vi "SAW.vi"(0 "File or Folder Path":path=path "G:/.shortcut-targets-by-id/0B8-gGFa6hkR4XzJJMDlqZXVKRk0/ansom/Data/MNK/SA40516Jref.20250417/05-Bsweepup", 5 "offset":i32, 7 "length":i32=400, 9 "index":T4={"S21"="S21", "S21 after subtraction"="S21", "S12"="S12", "S22"="S22", "Top gate "="frequency", "Bottom Gate"="frequency", "Local Gate"="frequency", "B/Time"="Magnet", "X axis"="frequency", "Temp"="Magnet Field"}, 11 "stop":bool, 12 "File Type":T3=enum."TDMS", 13 "decimate files":i32=2) -> (10 "Gates and B":T1={"Top gate"=100000000.0, "Bottom Gate"=100000000.0, "Local Gate"=100000000.0, "B"=0.11, "X axis"=100000000.0}, 14 "Comments":string="Device: \r  Device Name: SA40516Jref.20250417\r  Computer: Kholek\r  User: Muqing/Ranjani/Pubudu\r  Instrument: MNK\r  Description: |\r    KTO J Resonator - Reference\r    DC = 7/9 = KH1/2\r    Vbg=AO8=26\r\rExperiment: \r  Time: 2025-04-19T03:04:53\r  Description: |\r    T = 58mK\r    B=0T to 0.2T, 0.0005T step\r    Vbg(AO6) = 0V\r    Power: -19.6 dBm\r    0.1 to 2GHz\r    Vd: 1.3V\r    Id: 9.5mA\r\rSweep: \r- Loop1: [Magnet Field, 0.111000]\r- Loop2: [OFF, 0.000000]\r- Loop3: [OFF, 0.000000]\r- Loop4: [OFF, 0.000000]\r\rWiring: \r- Electrode 7: Lockin 1, I+\r- Electrode 11: Lockin 2, I-\r- Electrode 26: Lockin 8, \r\rLockin: \r  AO: \r  - AO 1: amp = 0.000 mV, DC = 0.000 mV, f = 13.00 Hz, phi = 0.00°, Sine\r  - AO 2: amp = 0.000 mV, DC = 0.000 mV, f = 13.00 Hz, phi = 0.00°, Sine\r  - AO 3: amp = 0.000 mV, DC = 0.000 mV, f = 13.00 Hz, phi = 0.00°, Sine\r  - AO 4: amp = 0.000 mV, DC = 0.000 mV, f = 13.00 Hz, phi = 0.00°, Sine\r  - AO 5: amp = 0.000 mV, DC = 0.000 mV, f = 13.00 Hz, phi = 0.00°, Sine\r  - AO 6: amp = 0.000 mV, DC = 0.000 mV, f = 13.00 Hz, phi = 0.00°, Sine\r  - AO 7: amp = 0.000 mV, DC = 0.000 mV, f = 13.00 Hz, phi = 0.00°, Sine\r  - AO 8: amp = 0.000 mV, DC = 0.000 mV, f = 13.00 Hz, phi = 0.00°, Sine\r  - AO 9: amp = 0.000 mV, DC = 0.000 mV, f = 13.00 Hz, phi = 0.00°, Sine\r  - AO 10: amp = 0.000 mV, DC = 0.000 mV, f = 13.00 Hz, phi = 0.00°, Sine\r  REF: \r  - Lockin 1: f = 13.00 Hz, phi = 0.00°, TC = 0.10 s, order = 2 \r  Sampling: \r  - Fs: 6500.000006\r  - N: 500\r")   [LabVIEW 2020]
uses:
  <userlib>/LevyLab/LV-Data/LV-Data/Typedefs/File Type--enum.ctl
  <userlib>/LevyLab/LV-Data/LV-Data/Typedefs/Dictionary--cluster.ctl
  <vilib>/Analysis/3filter.llb/Filter Passband Type.ctl
  <userlib>/LevyLab/Graph Utilities/graph_utilities.lvclass/graph_utilities.ctl
  <vilib>/Analysis/2dsp.llb/Decimate (single shot, DBL).vi
  <userlib>/LevyLab/XY Utilities/subVIs/Peak Detector (single).vi
  <userlib>/LevyLab/XY Utilities/subVIs/Subtract XY (single).vi
  <userlib>/LevyLab/XY Utilities/Private/X Units.vi
  <userlib>/LevyLab/XY Utilities/Private/X Array Range to Index.vi
  <userlib>/_MGI/1D Array/MGI Interpolate 1D Array Extended.vi
  <vilib>/Utility/error.llb/Error Cluster From Error Code.vi
  <vilib>/Analysis/3filter.llb/Butterworth Filter (DBL).vi
  <userlib>/LevyLab/Graph Utilities/graph_utilities.lvclass
  <userlib>/LevyLab/LV-Data/LV-Data/LV-Data.lvclass
  <vilib>/Analysis/NI_AALPro.lvlib
  <userlib>/LevyLab/XY Utilities/xy_utilities.lvlib
  <vilib>/Analysis/NI_AALBase.lvlib
panel:
  in  "Subtract this":cluster{dbl[], dbl[]}[](graph)=[{array[1601 elements], array[1601 elements]}]
  in  "filter order":i32=1
  in  "low cutoff freq":dbl=0.12500000000000006 format="%0.4f"
  in  "Add filter?":bool
  in  "Convert S21 to WAtts":bool
  out "XY-data out":cluster{"X-array":dbl[], "Y-array":dbl[]}[](array[cluster]) {"Y-array" format="%.2p"; "X-array" format="%.2p"}
  in  "threshold":dbl format="%0.2f"
  in  "width":dbl=3.0 min=3.0
  in  "Width Unit (points)":enum16{"Points", "Data"}(ring)
  out "Peak position vs parameter":cluster{dbl[], dbl[]}[](graph)
  out "S22":dbl[][](graph)
  out "S22 vs f":cluster{dbl[], dbl[]}[](graph)
  out "S12":dbl[][](graph)
  out "S12 vs f":cluster{dbl[], dbl[]}[](graph)
  out "S21 atr sub":dbl[][](graph)
  out "S11 vs f":cluster{dbl[], dbl[]}[](graph)
  out "S21":dbl[][](graph)
  in  "decimating factor":i32=1
  out "S21 vs f":cluster{dbl[], dbl[]}[](graph)
  out "Temp vs Field/Time":cluster{dbl[], dbl[]}[](graph)=[{[0.0001], [0.0]}, {[0.001], [0.001]}, {[0.002], [0.002]}, {[0.003], [0.003]}, {[0.004], [0.004]}, {[0.005], [0.005]}, {[0.006], [0.006]}, {[0.007], [0.007]}, {[0.008], [0.008]}, {[0.009], [0.009000000000000001]}, {[0.01], [0.01]}, {[0.011], [0.011]}, {[0.012], [0.012]}, {[0.013], [0.013000000000000001]}, {[0.014], [0.014]}, {[0.015], [0.015]}, {[0.016], [0.016]}, {[0.017], [0.017]}, {[0.018], [0.018000000000000002]}, {[0.019], [0.019]}, {[0.02], [0.02]}, {[0.021], [0.021]}, {[0.022], [0.022]}, {[0.0231], [0.023]}, {[0.024], [0.024]}, {[0.0251], [0.025]}, {[0.026], [0.026000000000000002]}, {[0.0269], [0.027]}, {[0.0281], [0.028]}, {[0.029], [0.029]}, {[0.03], [0.03]}, {[0.0311], [0.031]}, {[0.032], [0.032]}, {[0.033], [0.033]}, {[0.034], [0.034]}, {[0.035], [0.035]}, {[0.036], [0.036000000000000004]}, {[0.037], [0.037]}, {[0.0375], [0.038]}, {[0.039], [0.039]}, {[0.04], [0.04]}, {[0.041], [0.041]}, {[0.042], [0.042]}, {[0.043], [0.043000000000000003]}, {[0.044], [0.044]}, {[0.045], [0.045]}, {[0.046], [0.046]}, {[0.047], [0.047]}, {[0.048], [0.048]}, {[0.049], [0.049]}, {[0.05], [0.05]}, {[0.051], [0.051000000000000004]}, {[0.052], [0.052000000000000005]}, {[0.0527], [0.053]}, {[0.054], [0.054]}, {[0.055], [0.055]}, {[0.056], [0.056]}, {[0.057], [0.057]}, {[0.058], [0.058]}, {[0.059], [0.059000000000000004]}, {[0.06], [0.06]}, {[0.0611], [0.061]}, {[0.062], [0.062]}, {[0.063], [0.063]}, {[0.064], [0.064]}, {[0.065], [0.065]}, {[0.066], [0.066]}, {[0.0671], [0.067]}, {[0.068], [0.068]}, {[0.069], [0.069]}, {[0.07], [0.07]}, {[0.071], [0.07100000000000001]}, {[0.072], [0.07200000000000001]}, {[0.073], [0.073]}, {[0.074], [0.074]}, {[0.075], [0.075]}, {[0.076], [0.076]}, {[0.077], [0.077]}, {[0.078], [0.078]}, {[0.0791], [0.079]}, {[0.08], [0.08]}, {[0.081], [0.081]}, {[0.082], [0.082]}, {[0.083], [0.083]}, {[0.084], [0.084]}, {[0.085], [0.085]}, {[0.086], [0.08600000000000001]}, {[0.087], [0.08700000000000001]}, {[0.088], [0.088]}, {[0.089], [0.089]}, {[0.0901], [0.09]}, {[0.091], [0.091]}, {[0.092], [0.092]}, {[0.093], [0.093]}, {[0.094], [0.094]}, {[0.095], [0.095]}, {[0.096], [0.096]}, {[0.097], [0.097]}, {[0.098], [0.098]}, {[0.099], [0.099]}, {[0.1], [0.1]}, {[0.1011], [0.101]}, {[0.1019], [0.10200000000000001]}, {[0.103], [0.10300000000000001]}, {[0.104], [0.10400000000000001]}, {[0.105], [0.105]}, {[0.106], [0.106]}, {[0.107], [0.107]}, {[0.108], [0.108]}, {[0.1091], [0.109]}, {[0.11], [0.11]}, {[0.1111], [0.111]}, {[0.1121], [0.112]}, {[0.113], [0.113]}, {[0.114], [0.114]}, {[0.115], [0.115]}, {[0.116], [0.116]}, {[0.117], [0.117]}, {[0.118], [0.11800000000000001]}, {[0.119], [0.11900000000000001]}, {[0.12], [0.12]}, {[0.121], [0.121]}, {[0.122], [0.122]}, {[0.123], [0.123]}, {[0.124], [0.124]}, {[0.125], [0.125]}, {[0.126], [0.126]}, {[0.127], [0.127]}, {[0.128], [0.128]}, {[0.129], [0.129]}, {[0.13], [0.13]}, {[0.131], [0.131]}, {[0.132], [0.132]}, {[0.133], [0.133]}, {[0.134], [0.134]}, {[0.135], [0.135]}, {[0.136], [0.136]}, {[0.137], [0.137]}, {[0.138], [0.138]}, {[0.139], [0.139]}, {[0.14], [0.14]}, {[0.1411], [0.14100000000000001]}, {[0.142], [0.14200000000000002]}, {[0.143], [0.14300000000000002]}, {[0.144], [0.14400000000000002]}, {[0.1451], [0.145]}, {[0.146], [0.146]}, {[0.147], [0.147]}, {[0.1481], [0.148]}, {[0.149], [0.149]}, {[0.15], [0.15]}, {[0.151], [0.151]}, {[0.1521], [0.152]}, {[0.1531], [0.153]}, {[0.154], [0.154]}, {[0.155], [0.155]}, {[0.156], [0.156]}, {[0.157], [0.157]}, {[0.1581], [0.158]}, {[0.159], [0.159]}, {[0.1601], [0.16]}, {[0.161], [0.161]}, {[0.1621], [0.162]}, {[0.163], [0.163]}, {[0.164], [0.164]}, {[0.165], [0.165]}, {[0.166], [0.166]}, {[0.1671], [0.167]}, {[0.168], [0.168]}, {[0.169], [0.169]}, {[0.17], [0.17]}, {[0.171], [0.171]}, {[0.172], [0.17200000000000001]}, {[0.173], [0.17300000000000001]}, {[0.1741], [0.17400000000000002]}, {[0.175], [0.17500000000000002]}, {[0.176], [0.176]}, {[0.177], [0.177]}, {[0.178], [0.178]}, {[0.179], [0.179]}, {[0.1801], [0.18]}, {[0.1811], [0.181]}, {[0.182], [0.182]}, {[0.183], [0.183]}, {[0.184], [0.184]}, {[0.185], [0.185]}, {[0.186], [0.186]}, {[0.187], [0.187]}, {[0.188], [0.188]}, {[0.189], [0.189]}, {[0.19], [0.19]}, {[0.1911], [0.191]}, {[0.192], [0.192]}, {[0.193], [0.193]}, {[0.194], [0.194]}, {[0.195], [0.195]}, {[0.196], [0.196]}, {[0.197], [0.197]}, {[0.198], [0.198]}, {[0.1989], [0.199]}]
  in  "length":i32=10000
  in  "index":i32
  out "Data (Dictionary)":T2[](array[typedef])=[{"key"="OFF", "value"=variant(dbl[] [0.0])}, {"key"="Magnet Field", "value"=variant(dbl[] [0.111])}, {"key"="P", "value"=variant(dbl[] [-19.6])}, {"key"="Vds", "value"=variant(dbl[] [1.3])}, {"key"="Id", "value"=variant(dbl[] [9.5])}, {"key"="Vg", "value"=variant(dbl[] [0.0])}, {"key"="Temperature", "value"=variant(dbl[] [0.05700093922020847])}, {"key"="Magnet", "value"=variant(dbl[] [0.1111])}, {"key"="frequency", "value"=variant(dbl[] array[1601 elements])}, {"key"="ReS11", "value"=variant(dbl[] array[1601 elements])}, {"key"="ImS11", "value"=variant(dbl[] array[1601 elements])}, {"key"="ReS21", "value"=variant(dbl[] array[1601 elements])}, {"key"="ImS21", "value"=variant(dbl[] array[1601 elements])}, {"key"="ReS12", "value"=variant(dbl[] [])}, {"key"="ImS12", "value"=variant(dbl[] [])}, {"key"="ReS22", "value"=variant(dbl[] [])}, {"key"="ImS22", "value"=variant(dbl[] [])}, {"key"="S11", "value"=variant(dbl[] array[1601 elements])}, {"key"="S21", "value"=variant(dbl[] array[1601 elements])}, {"key"="S12", "value"=variant(dbl[] [])}, {"key"="S22", "value"=variant(dbl[] [])}]
  out "Path":path=path "G:/.shortcut-targets-by-id/0B8-gGFa6hkR4XzJJMDlqZXVKRk0/ansom/Data/MNK/SA40516Jref.20250417/05-Bsweepup/SA40516Jref.20250417.000222.tdms"
  out "counter":i32=111
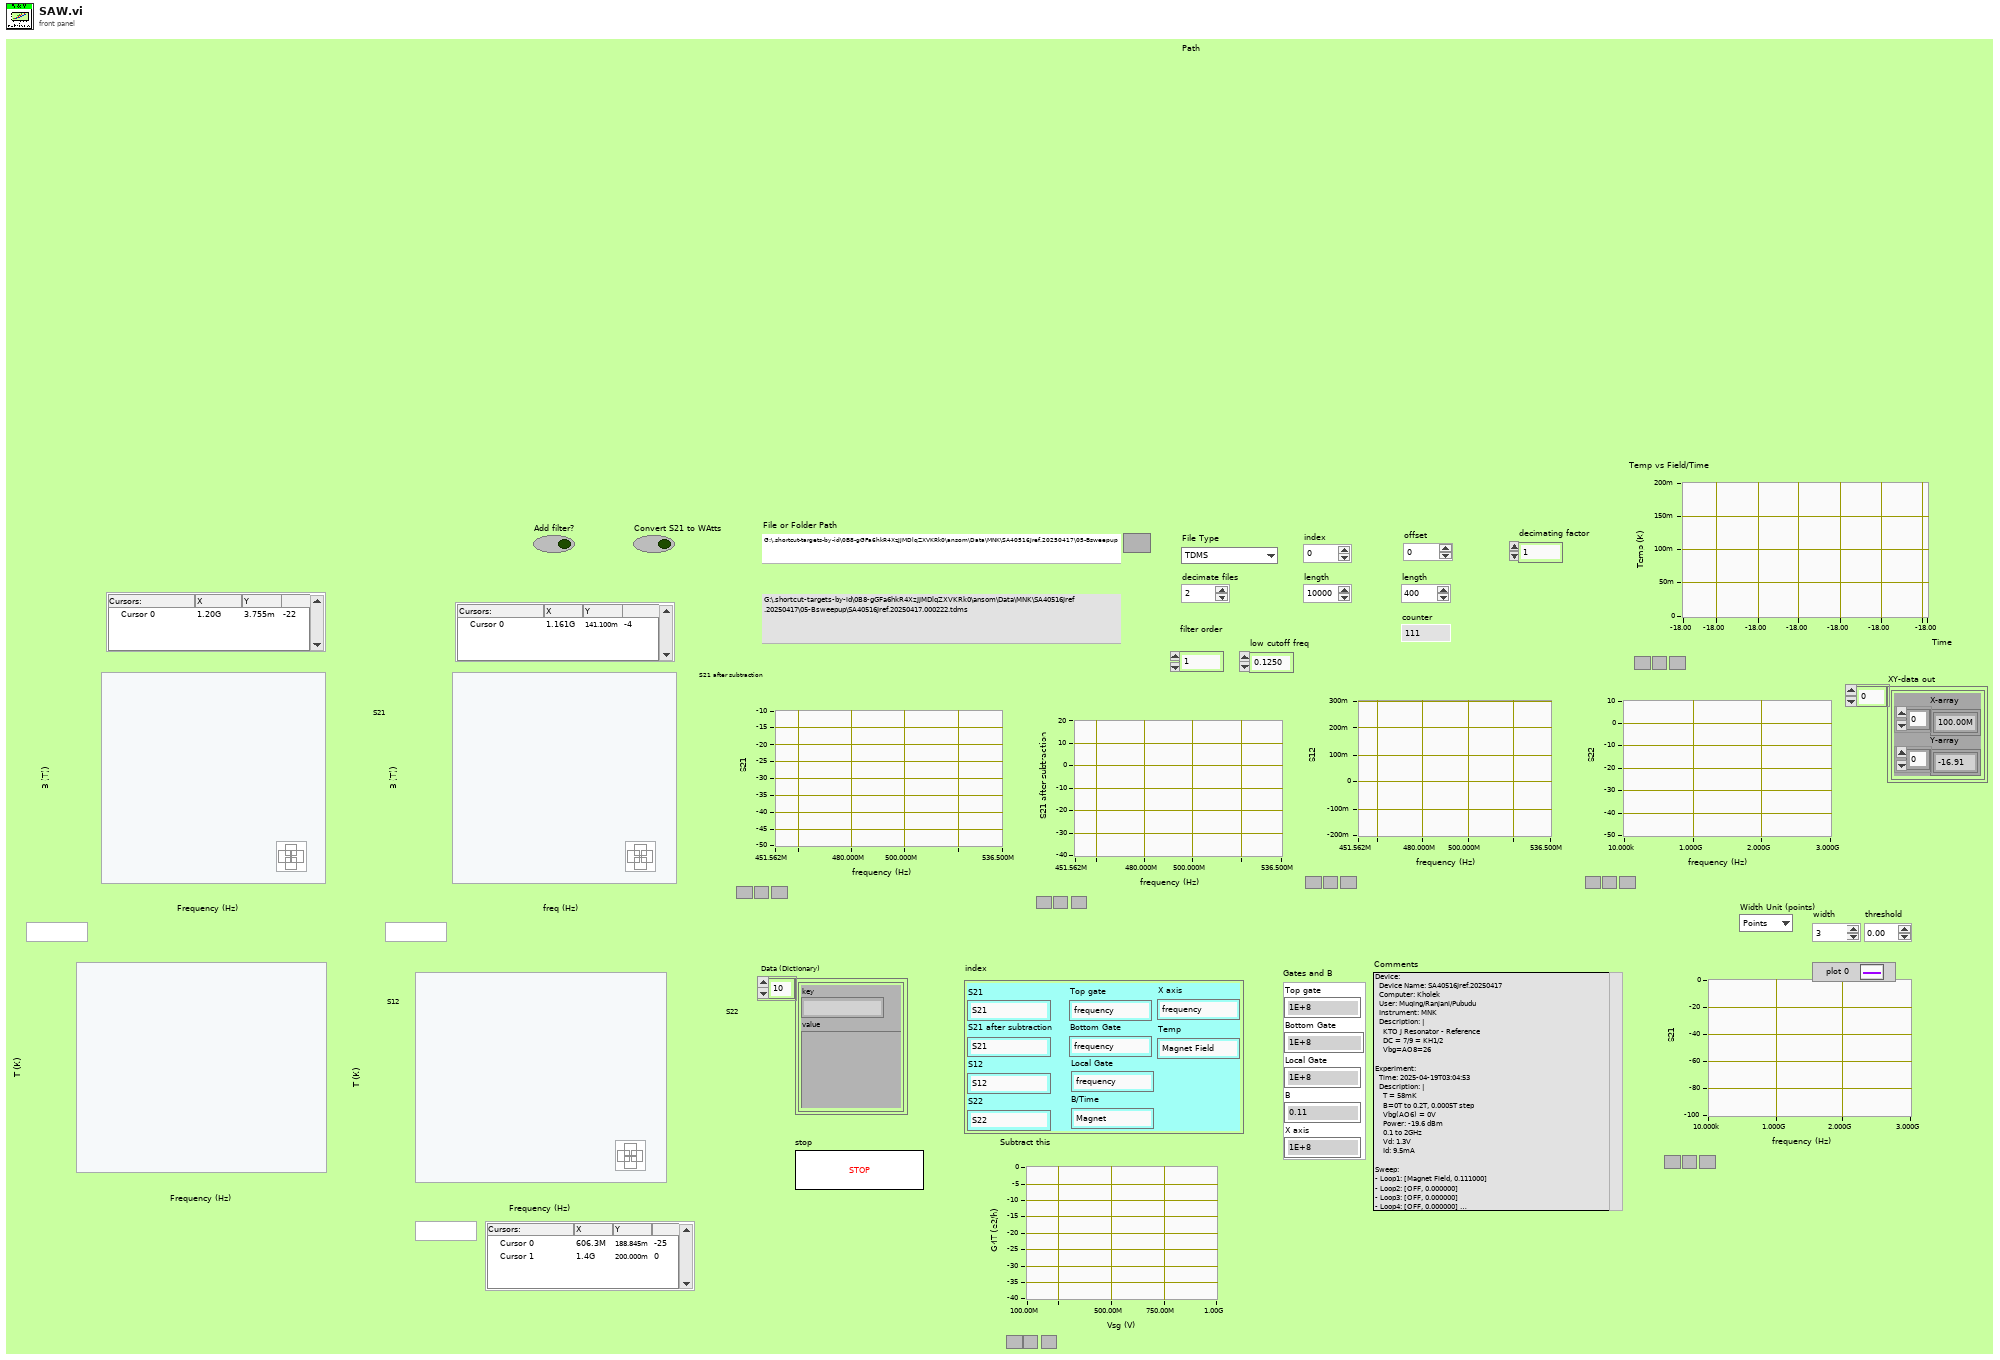
[diagram p1: front panel]
types:
  T1 = cluster{"Top gate":dbl, "Bottom Gate":dbl, "Local Gate":dbl, "B":dbl, "X axis":dbl}
  T2 = typedef "LV-Data.lvclass/Dictionary--cluster.ctl" = cluster{"key":string, "value":variant}
  T3 = typedef "LV-Data.lvclass/File Type--enum.ctl" = enum16{"DAT", "ITX", "TDMS", "VI"}
  T4 = cluster{"S21":string, "S21 after subtraction":string, "S12":string, "S22":string, "Top gate ":string, "Bottom Gate":string, "Local Gate":string, "B/Time":string, "X axis":string, "Temp":string}
  T5 = typedef "Dictionary Object RefNum__ogtk.ctl" = refnum<k1>
  T6 = typedef "NI_AALBase.lvlib/Filter Passband Type.ctl" = enum32{"Lowpass", "Highpass", "Bandpass", "Bandstop"}
  T7 = cluster{"Decimated Array":dbl[], "Decimated Array":dbl[]}
  T8 = cluster{"Decimated Array":dbl[], "Filtered X":dbl[]}
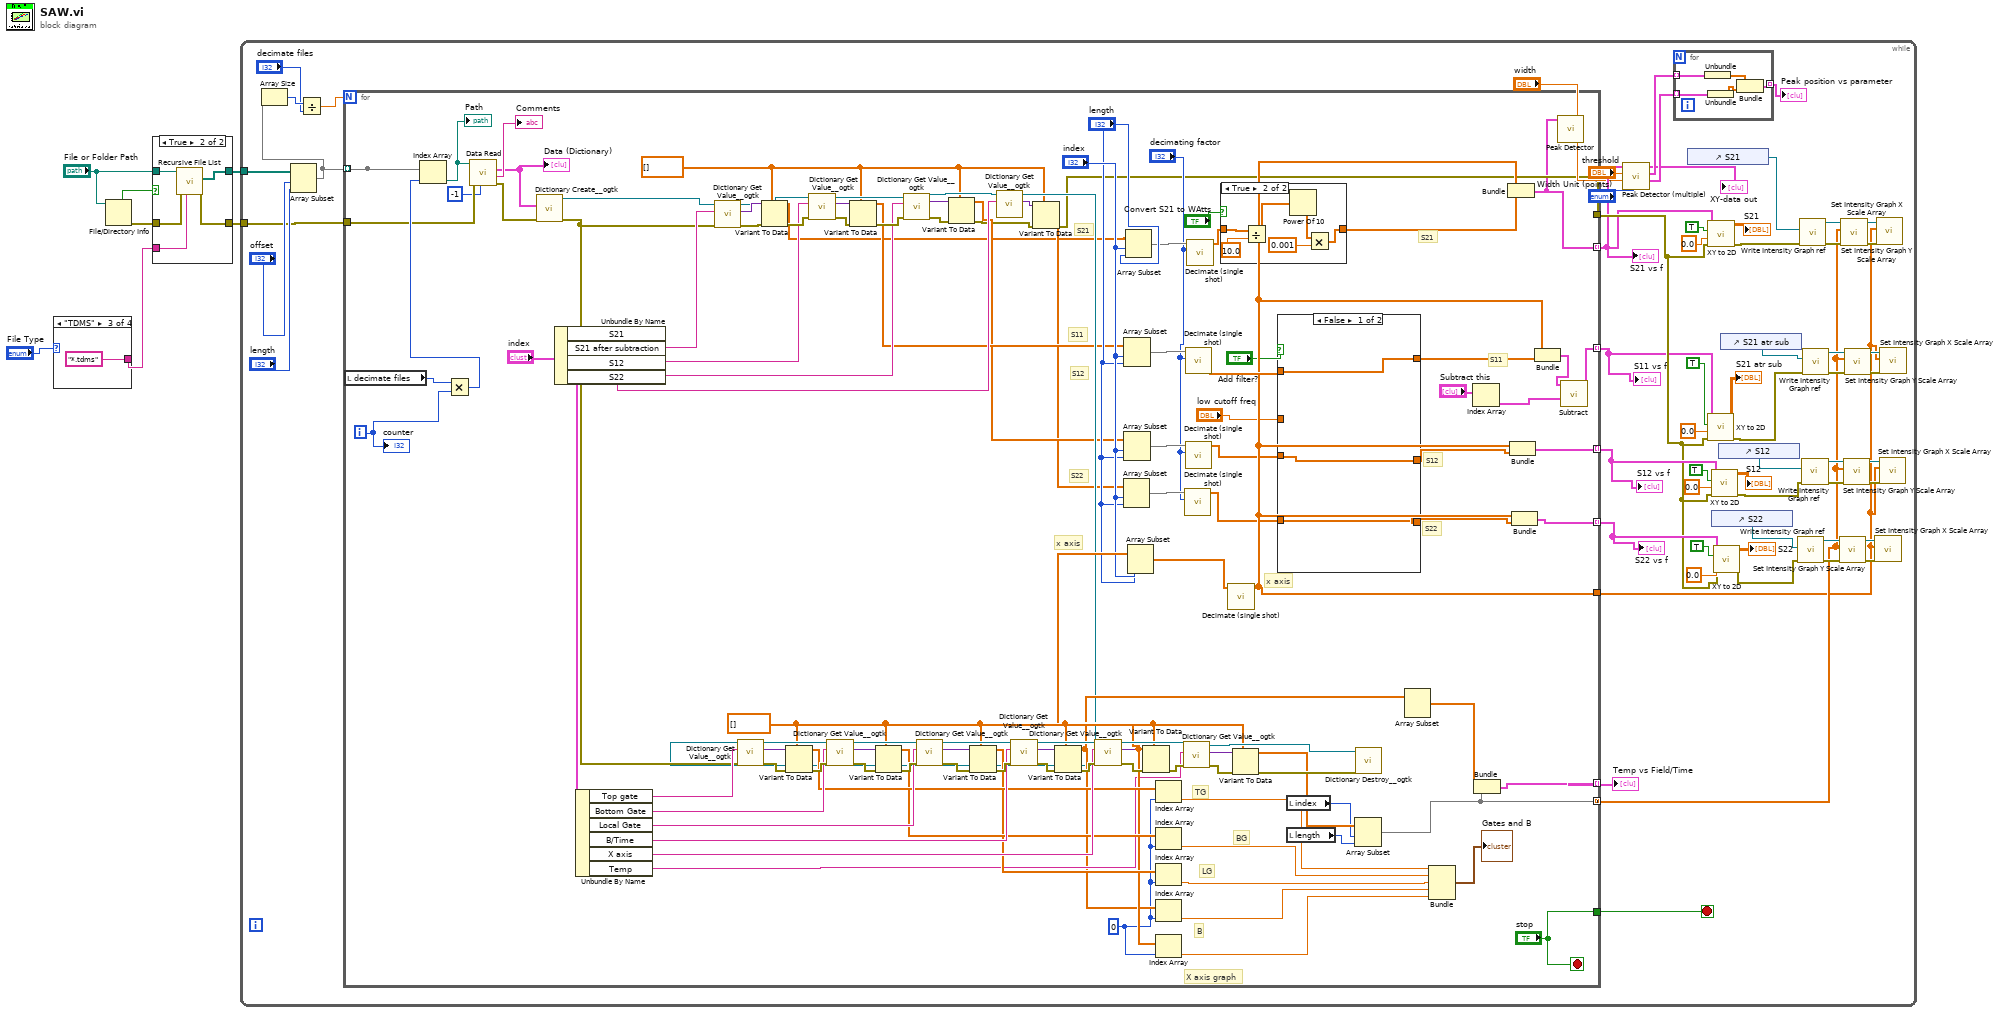
[diagram p0: block diagram]
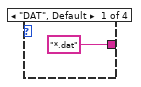
[diagram p2: hidden frame]
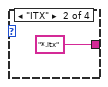
[diagram p3: hidden frame]
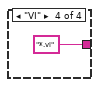
[diagram p4: hidden frame]
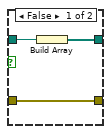
[diagram p5: hidden frame]
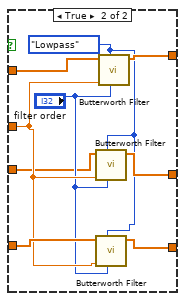
[diagram p6: hidden frame]
diagram:
  n1 = case shown="\"TDMS\"" "File Type" {
    tunnel: ["*.dat" ("pattern") "*.itx" ("pattern") "*.tdms" ("pattern") "*.vi" ("pattern")] -> w1
    frame "DAT", Default {
    }
    frame "ITX" {
    }
    frame "TDMS" {
    }
    frame "VI" {
    }
  }
  n2 = File/Directory Info(path="File or Folder Path") -> (directory=w5:bool, error out=w3:errorcluster)  [unwired: 1 in, 5 out]
  n3 = case shown="True" w5 {
    tunnel: [w14 w15] -> w6
    tunnel: "File or Folder Path" -> [w13 w19]
    tunnel: [w12 w18] -> w4
    tunnel: w3 -> [w12 w17]
    tunnel: w1 -> [_ w16]
    frame False {
      n4 = Build Array(w13) -> (w14:path[])
    }
    frame True {
      n5 = call <vilib>:"Recursive File List.vi"("pattern"=w16, "error in (no error)"=w17, "Folder Path"=w19) -> ("error out"=w18:errorcluster, "All Files in Dir"=w15:path[])  [unwired: 4 in, 3 out]
    }
  }
  n6 = while {
    tunnel: w6 -> [w77]
    tunnel: w4 -> [w72]
    stop <- w33 stop-if-true
    n7 = Array Subset(array=w77, index="offset", length="length") -> (w73:path[])
    n8 = Array Size(array=w73) -> (size(s)=w76:i32)
    n9 = Divide(x=w76, y="decimate files") -> (x/y=w74:dbl)
    n10 = for {
      N: w74 -> [_]
      tunnel: w73 -> [w198]
      tunnel: [w198] -> _ mode=indexing
      tunnel: w72 -> [w193]
      tunnel: [w98] -> w32 mode=indexing
      tunnel: [w132] -> w31 mode=indexing
      tunnel: [w85] -> w23 mode=indexing
      tunnel: [w105] -> w60 mode=indexing
      tunnel: [w104] -> w59 mode=indexing
      tunnel: [w102] -> w20
      tunnel: [w101] -> w21 mode=concatenating
      tunnel: [w100] -> w34
      tunnel: ["stop"] -> w33
      i -> [w195]
      stop <- "stop" stop-if-true
      w128 = 0 ("index")
      w139 = dbl[] []
      w114 = dbl[] []
      # "S22"
      # "S12"
      # "S11"
      # "S21"
      # "x axis"
      # "x axis"
      # "S22"
      # "S12"
      # "S11"
      # "S21"
      # "X axis graph"
      # "B"
      # "LG"
      # "BG"
      # "TG"
      n11 = local read "decimate files"() -> (w196:i32)
      n12 = Multiply(x=w196, y=w195) -> (x*y=w197:i32)
      n13 = Index Array(array=w198, index=w197) -> (element=w191:path)
      "Path" <- w191
      n14 = call <userlib>:"Data Read.vi"("Append Index"=-1, "error in (no error)"=w193, "path"=w191) -> ("error out"=w182:errorcluster, "Notes"=→"Comments":string, "Data (Dictionary)"=w190:T2[])  [unwired: 5 in, 1 out]
      "Data (Dictionary)" <- w190
      n15 = call <userlib>:"Dictionary Create__ogtk.vi"("error in (no error)"=w182, "initial dictionary (empty)"=w190) -> ("error out"=w145:errorcluster, "dictionary out"=w147:T5)  [unwired: 8 in]
      n16 = Unbundle By Name("index") -> ("S21"=w179:string, "S21 after subtraction"=w126:string, "S12"=w122:string, "S22"=w121:string)
      n17 = Unbundle By Name("index") -> ("Top gate"=w164:string, "Bottom Gate"=w163:string, "Local Gate"=w162:string, "B/Time"=w161:string, "X axis"=w156:string, "Temp"=w134:string)
      n18 = call <userlib>:"Dictionary Get Value__ogtk.vi"("error in"=w145, "key"=w179, "dictionary"=w147) -> ("error out"=w185:errorcluster, "value"=w184:variant, "dictionary out"=w183:T5)  [unwired: 5 in, 1 out]
      n19 = Variant To Data(error in=w185, type=w114, Variant=w184) -> (data=w107:dbl[], error out=w181:errorcluster)
      n20 = call <userlib>:"Dictionary Get Value__ogtk.vi"("error in"=w181, "key"=w126, "dictionary"=w183) -> ("error out"=w189:errorcluster, "value"=w188:variant, "dictionary out"=w152:T5)  [unwired: 5 in, 1 out]
      n21 = Variant To Data(error in=w189, type=w114, Variant=w188) -> (data=w118:dbl[], error out=w180:errorcluster)
      n22 = call <userlib>:"Dictionary Get Value__ogtk.vi"("error in"=w180, "key"=w122, "dictionary"=w152) -> ("error out"=w187:errorcluster, "value"=w186:variant, "dictionary out"=w125:T5)  [unwired: 5 in, 1 out]
      n23 = Variant To Data(error in=w187, type=w114, Variant=w186) -> (data=w117:dbl[], error out=w116:errorcluster)
      n24 = call <userlib>:"Dictionary Get Value__ogtk.vi"("key"=w121, "dictionary"=w125) -> ("value"=w123:variant, "dictionary out"=w124:T5)  [unwired: 6 in, 2 out]
      n25 = call <userlib>:"Dictionary Get Value__ogtk.vi"("error in"=w145, "key"=w164, "dictionary"=w124) -> ("error out"=w168:errorcluster, "value"=w178:variant, "dictionary out"=w171:T5)  [unwired: 5 in, 1 out]
      n26 = Variant To Data(error in=w168, type=w139, Variant=w178) -> (data=w155:dbl[], error out=w167:errorcluster)
      n27 = call <userlib>:"Dictionary Get Value__ogtk.vi"("error in"=w167, "key"=w163, "dictionary"=w171) -> ("error out"=w173:errorcluster, "value"=w172:variant, "dictionary out"=w170:T5)  [unwired: 5 in, 1 out]
      n28 = Variant To Data(error in=w173, type=w139, Variant=w172) -> (data=w154:dbl[], error out=w166:errorcluster)
      n29 = call <userlib>:"Dictionary Get Value__ogtk.vi"("error in"=w166, "key"=w162, "dictionary"=w170) -> ("error out"=w177:errorcluster, "value"=w176:variant, "dictionary out"=w169:T5)  [unwired: 5 in, 1 out]
      n30 = Variant To Data(error in=w177, type=w139, Variant=w176) -> (data=w146:dbl[], error out=w165:errorcluster)
      n31 = call <userlib>:"Dictionary Get Value__ogtk.vi"("error in"=w165, "key"=w161, "dictionary"=w169) -> ("error out"=w175:errorcluster, "value"=w174:variant, "dictionary out"=w158:T5)  [unwired: 5 in, 1 out]
      n32 = Variant To Data(error in=w116, type=w114, Variant=w123) -> (data=w115:dbl[], error out=w100:errorcluster)
      n33 = Variant To Data(error in=w175, type=w139, Variant=w174) -> (data=w129:dbl[], error out=w157:errorcluster)
      n34 = call <userlib>:"Dictionary Get Value__ogtk.vi"("error in"=w157, "key"=w156, "dictionary"=w158) -> ("error out"=w159:errorcluster, "value"=w160:variant, "dictionary out"=w143:T5)  [unwired: 5 in, 1 out]
      n35 = Array Subset(array=w115, index="index", length="length") -> (w110:dbl[])
      n36 = Array Subset(array=w118, index="index", length="length") -> (w112:dbl[])
      n37 = Array Subset(array=w117, index="index", length="length") -> (w111:dbl[])
      n38 = Array Subset(array=w107, index="index", length="length") -> (w113:dbl[])
      n39 = Variant To Data(error in=w159, type=w139, Variant=w160) -> (data=w136:dbl[], error out=w138:errorcluster)
      n40 = Array Subset(array=w136, index="index", length="length") -> (w127:dbl[])
      n41 = Index Array(array=w155, index=w128) -> (element=w151:dbl)
      n42 = Index Array(array=w154, index=w128) -> (element=w149:dbl)
      n43 = Index Array(array=w146, index=w128) -> (element=w150:dbl)
      n44 = Index Array(array=w129, index=w128) -> (element=w148:dbl)
      n45 = Index Array(array=w136, index=w128) -> (element=w144:dbl)
      n46 = call <userlib>:"Dictionary Get Value__ogtk.vi"("error in"=w138, "key"=w134, "dictionary"=w143) -> ("error out"=w137:errorcluster, "value"=w140:variant, "dictionary out"=w142:T5)  [unwired: 5 in, 1 out]
      n47 = call-poly <vilib>:"Decimate (single shot).vi"("decimating factor"="decimating factor", "X"=w110) -> ("Decimated Array"=w91:dbl[])  [unwired: 8 in, 1 out]
      n48 = call-poly <vilib>:"Decimate (single shot).vi"("decimating factor"="decimating factor", "X"=w112) -> ("Decimated Array"=w106:dbl[])  [unwired: 8 in, 1 out]
      n49 = call-poly <vilib>:"Decimate (single shot).vi"("decimating factor"="decimating factor", "X"=w111) -> ("Decimated Array"=w93:dbl[])  [unwired: 8 in, 1 out]
      n50 = call-poly <vilib>:"Decimate (single shot).vi"("decimating factor"="decimating factor", "X"=w113) -> ("Decimated Array"=w108:dbl[])  [unwired: 8 in, 1 out]
      n51 = case shown="True" "Convert S21 to WAtts" {
        tunnel: w108 -> [w211 w217]
        tunnel: [w211 w214] -> w97
        frame False {
        }
        frame True {
          n52 = Divide(x=w217, y=10.0) -> (x/y=w213:dbl[])
          n53 = Power Of 10(x=w213) -> (10^x=w215:dbl[])
          n54 = Multiply(x=w215, y=0.001) -> (x*y=w214:dbl[])
        }
      }
      n55 = call-poly <vilib>:"Decimate (single shot).vi"("X"=w127) -> ("Decimated Array"=w102:dbl[])  [unwired: 9 in, 1 out]
      n56 = Variant To Data(error in=w137, type=w139, Variant=w140) -> (data=w133:dbl[], error out=w135:errorcluster)
      n57 = case shown="False" "Add filter?" {
        tunnel: w106 -> [w201 w210]
        tunnel: [w201 w209] -> w95
        tunnel: w93 -> [w200 w202]
        tunnel: [w200 w208] -> w92
        tunnel: w91 -> [w199 w207]
        tunnel: [w199 w203] -> w90
        tunnel: "low cutoff freq" -> [_ w206]
        frame False {
        }
        frame True {
          w205 = Filter_Passband_Type."Lowpass" ("filter type")
          n58 = call-poly <vilib>:"Butterworth Filter.vi"("order"="filter order", "filter type"=w205, "low cutoff freq: fl"=w206, "X"=w202) -> ("Filtered X"=w208:dbl[])  [unwired: 4 in, 1 out]
          n59 = call-poly <vilib>:"Butterworth Filter.vi"("order"="filter order", "filter type"=w205, "low cutoff freq: fl"=w206, "X"=w207) -> ("Filtered X"=w203:dbl[])  [unwired: 4 in, 1 out]
          n60 = call-poly <vilib>:"Butterworth Filter.vi"("order"="filter order", "filter type"=w205, "low cutoff freq: fl"=w206, "X"=w210) -> ("Filtered X"=w209:dbl[])  [unwired: 4 in, 1 out]
        }
      }
      n61 = local read "index"() -> (w131:i32)
      n62 = local read "length"() -> (w130:i32)
      n63 = Array Subset(array=w133, index=w131, length=w130) -> (w101:dbl[])
      n64 = call <userlib>:"Dictionary Destroy__ogtk.vi"("error in (no error)"=w135, "dictionary"=w142) -> ()  [unwired: 9 in, 1 out]
      n65 = Array Subset(array=w129) -> (w103:dbl[])  [unwired: 2 in]
      n66 = Bundle(w151, w149, w150, w148, w144) -> (→"Gates and B":cluster{dbl, dbl, dbl, dbl, dbl})  [unwired: 1 in]
      n67 = Index Array(array="Subtract this") -> (element=w87:cluster{dbl[], dbl[]})  [unwired: 1 in]
      n68 = Bundle(w103, w101) -> (w132:cluster{dbl[], dbl[]})  [unwired: 1 in]
      n69 = Bundle("Decimated Array"=w102, "Decimated Array"=w97) -> (w98:T7)  [unwired: 1 in]
      n70 = Bundle("Decimated Array"=w102, "Filtered X"=w92) -> (w105:T8)  [unwired: 1 in]
      n71 = Bundle("Decimated Array"=w102, "Filtered X"=w90) -> (w104:T8)  [unwired: 1 in]
      n72 = Bundle("Decimated Array"=w102, "Filtered X"=w95) -> (w86:T8)  [unwired: 1 in]
      n73 = call-poly <vilib>:"Peak Detector.vi"("XY-data"=w98) -> ()  [unwired: 7 in, 4 out]
      n74 = call-poly <userlib>:"Subtract.vi"("y"=w87, "XY-data"=w86) -> ("XY-data out"=w85:cluster{"X-array":dbl[], "Y-array":dbl[]})  [unwired: 8 in, 1 out]
      "counter" <- w195
    }
    "Temp vs Field/Time" <- w31
    "S21 vs f" <- w32
    "S11 vs f" <- w23
    "S12 vs f" <- w60
    "S22 vs f" <- w59
    n75 = call <userlib>:"Peak Detector (multiple).vi"("Width Unit (points)"="Width Unit (points)", "width"="width", "threshold"="threshold", "XY-data"=w32) -> ("Amplitudes"=w29:cluster{"Amplitudes":dbl[]}[], "Locations"=w30:cluster{"Locations":dbl[]}[], "XY-data out"=→"XY-data out":cluster{"X-array":dbl[], "Y-array":dbl[]}[])  [unwired: 4 in, 1 out]
    n76 = for {
      tunnel: w30 -> [w84] mode=indexing
      tunnel: w29 -> [w83] mode=indexing
      tunnel: [w80] -> w28 mode=indexing
      n77 = Unbundle(w84) -> ("Locations"=w82:dbl[])
      n78 = Unbundle(w83) -> ("Amplitudes"=w81:dbl[])
      n79 = Bundle("Locations"=w82, "Amplitudes"=w81) -> (w80:cluster{"Locations":dbl[], "Amplitudes":dbl[]})  [unwired: 1 in]
    }
    "Peak position vs parameter" <- w28
    n80 = control-ref of="S21"() -> (w58:refnum<vi>)
    n81 = call <userlib>:"XY to 2D.vi"("error in (no error)"=w34, "Fake Point"=0.0, "Interpolate [T]"=TRUE, "XY-data"=w23) -> ("error out"=w37:errorcluster, "2D Y Array"=→"S21 atr sub":dbl[][])  [unwired: 4 in, 2 out]
    n82 = call <userlib>:"XY to 2D.vi"("error in (no error)"=w34, "Fake Point"=0.0, "Interpolate [T]"=TRUE, "XY-data"=w32) -> ("error out"=w40:errorcluster, "2D Y Array"=→"S21":dbl[][])  [unwired: 4 in, 2 out]
    n83 = call <userlib>:"XY to 2D.vi"("error in (no error)"=w34, "Fake Point"=0.0, "Interpolate [T]"=TRUE, "XY-data"=w60) -> ("error out"=w35:errorcluster, "2D Y Array"=→"S12":dbl[][])  [unwired: 4 in, 2 out]
    n84 = control-ref of="S22"() -> (w43:refnum<vi>)
    n85 = call <userlib>:"XY to 2D.vi"("error in (no error)"=w34, "Fake Point"=0.0, "Interpolate [T]"=TRUE, "XY-data"=w59) -> ("error out"=w39:errorcluster, "2D Y Array"=→"S22":dbl[][])  [unwired: 4 in, 2 out]
    n86 = control-ref of="S12"() -> (w44:refnum<vi>)
    n87 = control-ref of="S21 atr sub"() -> (w45:refnum<vi>)
    n88 = call <userlib>:"Write Intensity Graph ref.vi"("error in (no error)"=w39, "Intensity Graph"=w43) -> ("error out"=w41:errorcluster, "graph_utilities out"=w48:refnum<class "graph_utilities.lvclass">)  [unwired: 8 in]
    n89 = call <userlib>:"Write Intensity Graph ref.vi"("error in (no error)"=w40, "Intensity Graph"=w58) -> ("error out"=w38:errorcluster, "graph_utilities out"=w57:refnum<class "graph_utilities.lvclass">)  [unwired: 8 in]
    n90 = call <userlib>:"Write Intensity Graph ref.vi"("error in (no error)"=w35, "Intensity Graph"=w44) -> ("error out"=w42:errorcluster, "graph_utilities out"=w51:refnum<class "graph_utilities.lvclass">)  [unwired: 8 in]
    n91 = call <userlib>:"Write Intensity Graph ref.vi"("error in (no error)"=w37, "Intensity Graph"=w45) -> ("error out"=w36:errorcluster, "graph_utilities out"=w54:refnum<class "graph_utilities.lvclass">)  [unwired: 8 in]
    n92 = call <userlib>:"Set Intensity Graph Y Scale Array.vi"("error in (no error)"=w41, "Y Scale"=w21, "graph_utilities in"=w48) -> ("error out"=w47:errorcluster, "graph_utilities out"=w46:refnum<class "graph_utilities.lvclass">)  [unwired: 7 in]
    n93 = call <userlib>:"Set Intensity Graph Y Scale Array.vi"("error in (no error)"=w38, "Y Scale"=w21, "graph_utilities in"=w57) -> ("error out"=w56:errorcluster, "graph_utilities out"=w55:refnum<class "graph_utilities.lvclass">)  [unwired: 7 in]
    n94 = call <userlib>:"Set Intensity Graph Y Scale Array.vi"("error in (no error)"=w42, "Y Scale"=w21, "graph_utilities in"=w51) -> ("error out"=w50:errorcluster, "graph_utilities out"=w49:refnum<class "graph_utilities.lvclass">)  [unwired: 7 in]
    n95 = call <userlib>:"Set Intensity Graph Y Scale Array.vi"("error in (no error)"=w36, "Y Scale"=w21, "graph_utilities in"=w54) -> ("error out"=w53:errorcluster, "graph_utilities out"=w52:refnum<class "graph_utilities.lvclass">)  [unwired: 7 in]
    n96 = call <userlib>:"Set Intensity Graph X Scale Array.vi"("error in (no error)"=w47, "X Scale"=w20, "graph_utilities in"=w46) -> ()  [unwired: 7 in, 2 out]
    n97 = call <userlib>:"Set Intensity Graph X Scale Array.vi"("error in (no error)"=w56, "X Scale"=w20, "graph_utilities in"=w55) -> ()  [unwired: 7 in, 2 out]
    n98 = call <userlib>:"Set Intensity Graph X Scale Array.vi"("error in (no error)"=w50, "X Scale"=w20, "graph_utilities in"=w49) -> ()  [unwired: 7 in, 2 out]
    n99 = call <userlib>:"Set Intensity Graph X Scale Array.vi"("error in (no error)"=w53, "X Scale"=w20, "graph_utilities in"=w52) -> ()  [unwired: 7 in, 2 out]
  }
